vi "Get Minimum dt.vi"(0 "Instrument handle IN":refnum<k15>[](array[refnum]), 5 "Channel Name":string[](array[string]), 11 "error in (no error)":errorcluster) -> (4 "Instrument handle OUT":refnum<k15>[](array[refnum]), 6 "Minimum dt":dbl[](array[numeric]), 15 "error out":errorcluster)   [LabVIEW 2024, in "devicePowerSequencerCoreLogic.lvlib"]
uses:
  devicePowerSequencerCoreLogic.lvlib
  <instrlib>/niDCPower/nidcpower.llb/niDCPower Sequence Attribute Type.ctl
  <vilib>/Utility/config.llb/Read Key (Double).vi
  <instrlib>/niDCPower/nidcpower.llb/niDCPower Create Advanced Sequence Step With Channels.vi
  <vilib>/Utility/config.llb/NI_LVConfig.lvlib
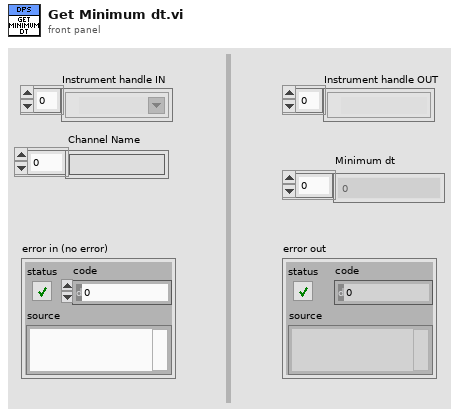
[diagram p1: front panel]
types:
  T1 = typedef "NI_LVConfig.lvlib/Config Data RefNum.ctl" = refnum<k1>
  T2 = typedef "niDCPower Sequence Attribute Type.ctl" = i32
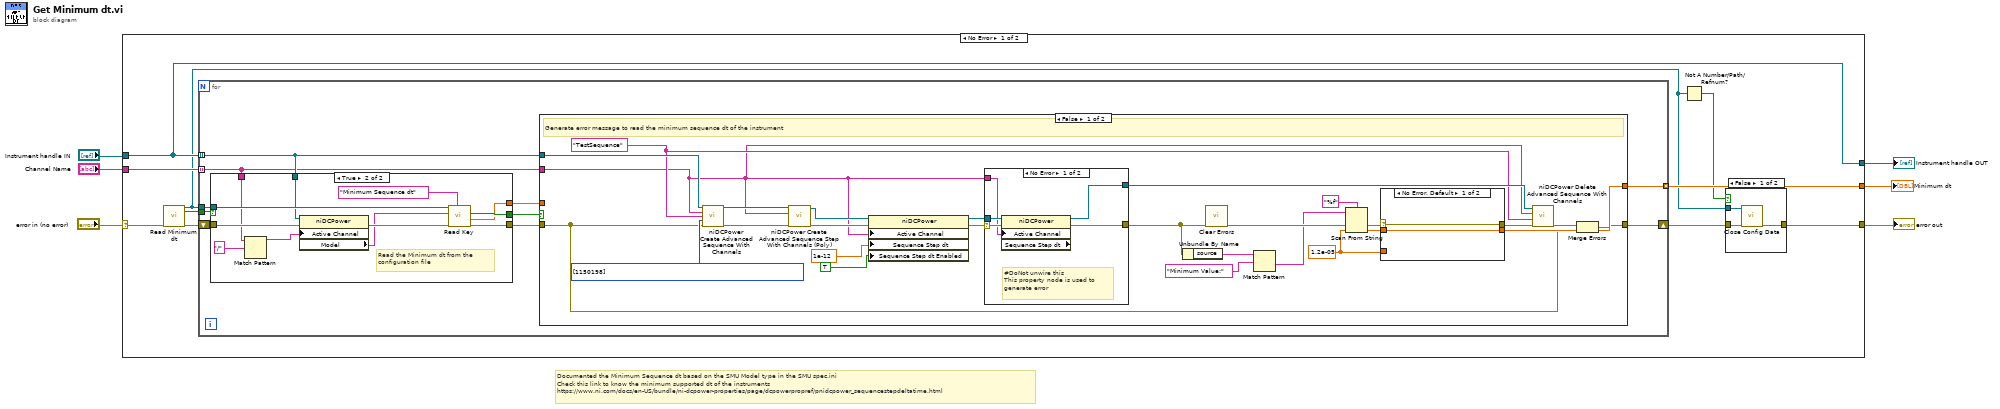
[diagram p0: block diagram]
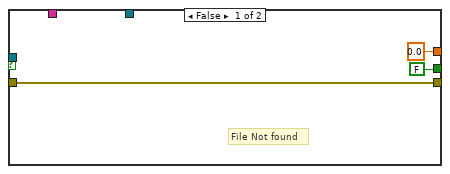
[diagram p3: hidden frame]
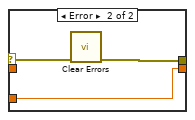
[diagram p4: hidden frame]
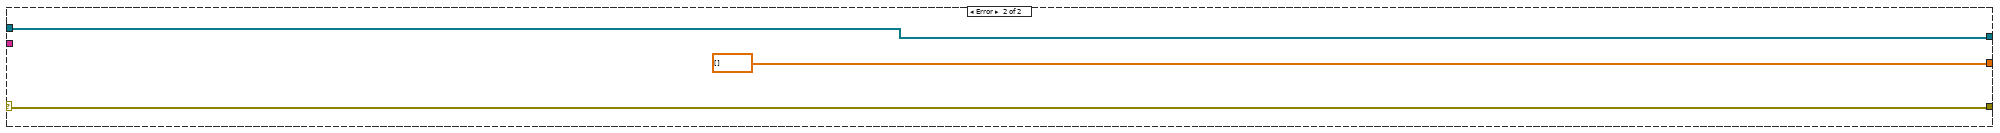
[diagram p7: hidden frame]
diagram:
  # "Documented the Minimum Sequence dt based on the SMU Model type in the SMU spec.ini\nCheck this link to know the minimum supported dt of the instruments\nhttps://www.ni.com/docs/en-US/bundle/ni-dcpower-properties/page/dcpowerpropref/pnidcpower_sequencestepdeltatime.html"
  n1 = case shown="No Error" "error in (no error)" {
    selector: "error in (no error)" -> [w14 w89]
    tunnel: "Instrument handle IN" -> [w15 w87]
    tunnel: [w11 w89] -> w4
    tunnel: [w16 dbl[] []] -> w3
    tunnel: [w15 w87] -> w2
    tunnel: "Channel Name" -> [w10 _]
    frame No Error {
      n2 = call "Read Minimum dt.vi"("error in (no error)"=w14) -> ("refnum"=w7:T1, "File Exist?"=w9:bool, "error out"=w13:errorcluster)  [unwired: 12 in]
      n3 = for {
        tunnel: w15 -> [w27] mode=indexing
        tunnel: [w25] -> w16 mode=indexing
        shift-right: [w24] -> w12
        shift-left: w13 -> [w29]
        tunnel: w7 -> [w30]
        tunnel: w10 -> [w22] mode=indexing
        tunnel: w9 -> [w23]
        n4 = case shown="True" w23 {
          tunnel: w30 -> [_ w45]
          tunnel: w29 -> [w33 w43]
          tunnel: [w33 w41] -> w28
          tunnel: [FALSE ("found?") w40] -> w21
          tunnel: w27 -> [_ w39]
          tunnel: [0.0 ("value") w38] -> w26
          tunnel: w22 -> [_ w36]
          frame False {
            # "File Not found"
          }
          frame True {
            # "Read the Minimum dt from the\nconfiguration file"
            n5 = Match Pattern(string=w36, regular expression="/") -> (before substring=w34:string)  [unwired: 1 in, 3 out]
            n6 = property class="niDCPower"(reference=w39, error in=w43, "Active Channel"=w34) -> (error out=w42:errorcluster, "Model"=w37:string)  [unwired: 1 out]
            n7 = call-poly <vilib>:"Read Key.vi"("section"="Minimum Sequence dt", "error in (no error)"=w42, "key"=w37, "refnum"=w45) -> ("error out"=w41:errorcluster, "value"=w38:dbl, "found?"=w40:bool)  [unwired: 4 in, 1 out]
          }
        }
        n8 = case shown="False" w21 {
          tunnel: w28 -> [w46 w85]
          tunnel: w27 -> [w69 _]
          tunnel: w26 -> [_ w86]
          tunnel: [w47 w85] -> w24
          tunnel: [w51 w86] -> w25
          tunnel: w22 -> [w48 _]
          frame False {
            w50 = 1.2e-05 ("default value 1")
            w60 = "TestSequence" ("sequence name")
            w72 = T2[] [1150198] items=["Source -> Output Function"=1150008, "Source -> Output Enabled"=1250006, "Source -> Output Resistance"=1150061, "Source -> Transient Response"=1150062, "Source -> Custom Transient Response -> Voltage Gain Bandwidth"=1150067, "Source -> Custom Transient Response -> Voltage Compensation Frequency"=1150068, "Source -> Custom Transient Response -> Voltage Pole-Zero Ratio"=1150069, "Source -> Custom Transient Response -> Current Gain Bandwidth"=1150070, "Source -> Custom Transient Response -> Current Compensation Frequency"=1150071, "Source -> Custom Transient Response -> Current Pole-Zero Ratio"=1150072, "Source -> DC Voltage -> Voltage Level"=1250001, "Source -> DC Voltage -> Voltage Level Range"=1150005, "Source -> DC Voltage -> Current Limit"=1250005, "Source -> DC Voltage -> Current Limit High"=1150187, "Source -> DC Voltage -> Current Limit Low"=1150188, "Source -> DC Voltage -> Current Limit Range"=1150004, "Source -> DC Current -> Current Level"=1150009, "Source -> DC Current -> Current Level Range"=1150011, "Source -> DC Current -> Voltage Limit"=1150010, "Source -> DC Current -> Voltage Limit High"=1150185, "Source -> DC Current -> Voltage Limit Low"=1150186, "Source -> DC Current -> Voltage Limit Range"=1150012, "Source -> Pulse Voltage -> Pulse Voltage Level"=1150080, "Source -> Pulse Voltage -> Pulse Bias Voltage Level"=1150082, "Source -> Pulse Voltage -> Pulse Voltage Level Range"=1150084, "Source -> Pulse Voltage -> Pulse Current Limit"=1150081, "Source -> Pulse Voltage -> Pulse Current Limit High"=1150193, "Source -> Pulse Voltage -> Pulse Current Limit Low"=1150194, "Source -> Pulse Voltage -> Pulse Bias Current Limit"=1150083, "Source -> Pulse Voltage -> Pulse Bias Current Limit High"=1150195, "Source -> Pulse Voltage -> Pulse Bias Current Limit Low"=1150196, "Source -> Pulse Voltage -> Pulse Current Limit Range"=1150085, "Source -> Pulse Current -> Pulse Current Level"=1150086, "Source -> Pulse Current -> Pulse Bias Current Level"=1150088, "Source -> Pulse Current -> Pulse Current Level Range"=1150090, "Source -> Pulse Current -> Pulse Voltage Limit"=1150087, "Source -> Pulse Current -> Pulse Voltage Limit High"=1150189, "Source -> Pulse Current -> Pulse Voltage Limit Low"=1150190, "Source -> Pulse Current -> Pulse Bias Voltage Limit"=1150089, "Source -> Pulse Current -> Pulse Bias Voltage Limit High"=1150191, "Source -> Pulse Current -> Pulse Bias Voltage Limit Low"=1150192, "Source -> Pulse Current -> Pulse Voltage Limit Range"=1150091, "Source -> Advanced -> Source Delay"=1150051, "Source -> Advanced -> Pulse Bias Delay"=1150092, "Source -> Advanced -> Pulse On Time"=1150093, "Source -> Advanced -> Pulse Off Time"=1150094, "Source -> Advanced -> OVP Enabled"=1250002, "Source -> Advanced -> OVP Limit"=1250003, "Source -> Advanced -> Compliance Limit Symmetry"=1150184, "Source -> Advanced -> Sequence Step Delta Time"=1150198, "Measurement -> Sense"=1150013, "Measurement -> Aperture Time"=1150058, "Measurement -> Measure Record Length"=1150063, "Measurement -> Advanced -> DC Noise Rejection"=1150066, "Measurement -> Autorange"=1150244, "Measurement -> Advanced -> Autorange Behavior"=1150245, "Measurement -> Advanced -> Autorange Aperture Time Mode"=1150246, "Measurement -> Advanced -> Autorange Minimum Aperture Time"=1150247, "Measurement -> Advanced -> Autorange Minimum Aperture Time Units"=1150248, "Measurement -> Advanced -> Autorange Minimum Current Range"=1150255, "Measurement -> Advanced -> Autorange Minimum Voltage Range"=1150256, "Measurement -> Advanced -> Autorange Threshold Mode"=1150257, "Measurement -> Advanced -> Autorange Maximum Delay After Range Change"=1150322, "LCR -> Instrument Mode"=1150208, "LCR -> Source Delay Mode"=1150315, "LCR -> Measurement Time"=1150218, "LCR -> Custom Measurement Time"=1150258, "LCR -> AC Stimulus -> Function"=1150209, "LCR -> AC Stimulus -> Frequency"=1150210, "LCR -> AC Stimulus -> Voltage Amplitude"=1150211, "LCR -> AC Stimulus -> Current Amplitude"=1150212, "LCR -> AC Stimulus -> Advanced -> Voltage Range"=1150265, "LCR -> AC Stimulus -> Advanced -> Current Range"=1150267, "LCR -> DC Bias -> Source"=1150213, "LCR -> DC Bias -> Voltage Level"=1150214, "LCR -> DC Bias -> Current Level"=1150215, "LCR -> DC Bias -> Advanced -> Voltage Range"=1150266, "LCR -> DC Bias -> Advanced -> Current Range"=1150274, "LCR -> Compensation -> Open -> Enabled"=1150220, "LCR -> Compensation -> Open -> Conductance"=1150261, "LCR -> Compensation -> Open -> Susceptance"=1150262, "LCR -> Compensation -> Short -> Enabled"=1150221, "LCR -> Compensation -> Short -> Resistance"=1150263, "LCR -> Compensation -> Short -> Reactance"=1150264, "LCR -> Compensation -> Load -> Enabled"=1150222, "LCR -> Compensation -> Load -> Measured Resistance"=1150268, "LCR -> Compensation -> Load -> Measured Reactance"=1150269, "LCR -> Compensation -> Load -> Actual Resistance"=1150270, "LCR -> Compensation -> Load -> Actual Reactance"=1150271, "LCR -> Impedance Range -> Impedance Range"=1150217, "LCR -> Impedance Range -> Impedance Autorange"=1150216, "LCR -> Impedance Range -> Advanced -> Impedance Range Source"=1150321, "LCR -> Impedance Range -> Advanced -> Load Resistance"=1150318, "LCR -> Impedance Range -> Advanced -> Load Inductance"=1150319, "LCR -> Impedance Range -> Advanced -> Load Capacitance"=1150320] ("advanced sequence properties")
            # "Generate error message to read the minimum sequence dt of the instrument"
            n9 = call <instrlib>:"niDCPower Create Advanced Sequence With Channels.vi"("instrument handle"=w69, "channel name"=w48, "sequence name"=w60, "advanced sequence properties"=w72, "error in (no error)"=w46) -> ("instrument handle out"=w70:refnum<k15>, "error out"=w71:errorcluster)  [unwired: 9 in]
            n10 = call-poly <instrlib>:"niDCPower Create Advanced Sequence Step With Channels (Poly).vi"("error in (no error)"=w71, "channel name"=w48, "instrument handle"=w70) -> ("error out"=w67:errorcluster, "instrument handle out"=w68:refnum<k15>)  [unwired: 7 in]
            n11 = property class="niDCPower"(reference=w68, error in=w67, "Active Channel"=w48, "Sequence Step dt"=1e-12 ("Source:Advanced:Sequence Step Delta Time"), "Sequence Step dt Enabled"=TRUE ("Source:Advanced:Sequence Step Delta Time Enabled")) -> (reference out=w64:refnum<k15>, error out=w65:errorcluster)
            n12 = case shown="No Error" w65 {
              selector: w65 -> [w81 w84]
              tunnel: w64 -> [w82 w83]
              tunnel: [w80 w84] -> w58
              tunnel: [w79 w83] -> w61
              tunnel: w48 -> [w78 _]
              frame No Error {
                # "#DoNot unwire this\nThis property node is used to \ngenerate error"
                n13 = property class="niDCPower" props=["Active Channel", "Sequence Step dt"](reference=w82, error in=w81, "Active Channel"=w78) -> (reference out=w79:refnum<k15>, error out=w80:errorcluster)  [unwired: 1 out]
              }
              frame Error {
              }
            }
            n14 = Unbundle By Name(w58) -> ("source"=w57:string)
            n15 = call <vilib>:"Clear Errors.vi"("error in (no error)"=w58) -> ("error out"=w63:errorcluster)  [unwired: 5 in, 1 out]
            n16 = Match Pattern(string=w57, regular expression="Minimum Value:") -> (after substring=w56:string)  [unwired: 1 in, 3 out]
            n17 = Scan From String(format string="%f", input string=w56, error in=w63, default 1=w50) -> (error out=w54:errorcluster, output 1=w52:dbl)  [unwired: 1 in, 2 out]
            n18 = case shown="No Error, Default" w54 {
              selector: w54 -> [w73 w77]
              tunnel: [w73 w76] -> w53
              tunnel: w52 -> [w74 _]
              tunnel: [w74 w75] -> w51
              tunnel: w50 -> [_ w75]
              frame No Error {
              }
              frame Error {
                n19 = call <vilib>:"Clear Errors.vi"("error in (no error)"=w77) -> ("error out"=w76:errorcluster)  [unwired: 5 in, 1 out]
              }
            }
            n20 = call <instrlib>:"niDCPower Delete Advanced Sequence With Channels.vi"("error in (no error)"=w53, "sequence name"=w60, "channel name"=w48, "instrument handle"=w61) -> ("error out"=w59:errorcluster)  [unwired: 6 in, 1 out]
            n21 = Merge Errors(w59, w46) -> (w47:errorcluster)
          }
          frame True {
            # "Minimum dt is found in the configuration File"
          }
        }
      }
      n22 = Not A Number/Path/Refnum?(number/path/refnum=w7) -> (NaN/Path/Refnum?=w8:bool)
      n23 = case shown="False" w8 {
        tunnel: w12 -> [w19 w20]
        tunnel: [w18 w20] -> w11
        tunnel: w7 -> [w17 _]
        frame False {
          n24 = call <vilib>:"Close Config Data.vi"("error in (no error)"=w19, "refnum"=w17) -> ("error out"=w18:errorcluster)  [unwired: 8 in, 1 out]
        }
        frame True {
        }
      }
    }
    frame Error {
    }
  }
  "error out" <- w4
  "Instrument handle OUT" <- w2
  "Minimum dt" <- w3
